vi "Remove Sequence Element.vi"(8 "error in (no error)":errorcluster, 10 "Name":string, 11 "Sequence Controller in":refnum<class "Sequence Controller.lvclass">) -> (0 "error out":errorcluster, 3 "Sequence Controller out":refnum<class "Sequence Controller.lvclass">)   [LabVIEW 2016, in "Sequence Controller.lvclass"]
uses:
  Sequence Controller.lvclass
  C:/Program Files/National Instruments/LabVIEW 2016/vi.lib/ActorFramework/Actor/Actor.lvclass
  <vilib>/ActorFramework/Actor/Actor.lvclass/Actor.ctl
  Sequence Controller.lvclass/Sequence Controller.ctl
  Template Module Messages/Stop Object Msg/Stop Object Msg.lvclass/Stop Object Msg.ctl
  <vilib>/ActorFramework/Message Enqueuer/Message Enqueuer.lvclass/Message Enqueuer.ctl
  <vilib>/ActorFramework/Message Enqueuer/Enqueue.vi
  Template Module Messages/Stop Object Msg/Stop Object Msg.lvclass
  C:/Program Files/National Instruments/LabVIEW 2016/vi.lib/ActorFramework/Message/Message.lvclass
  <vilib>/ActorFramework/Message Priority Queue/Priority Enqueue.vi
  <vilib>/ActorFramework/Actor/Actor.lvclass
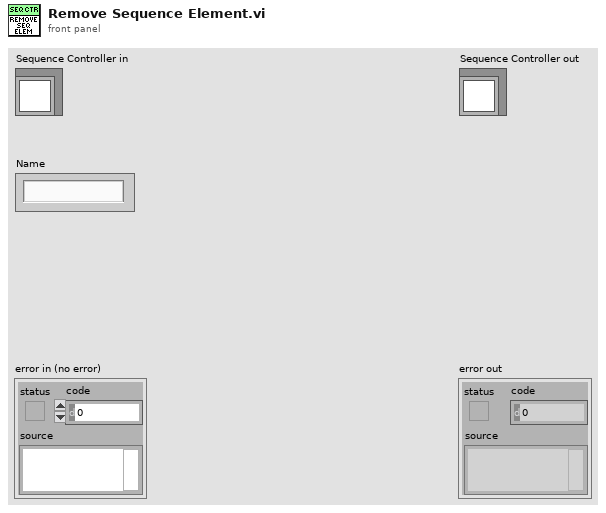
[diagram p1: front panel]
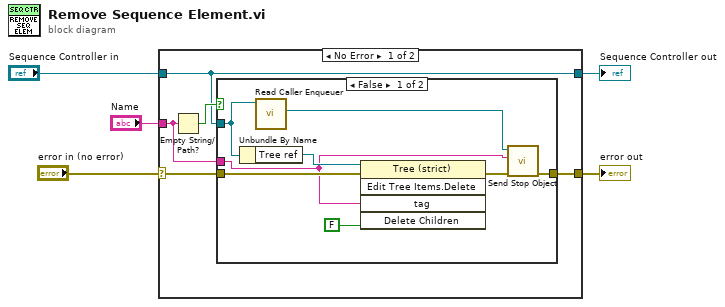
[diagram p0: block diagram]
diagram:
  n1 = case shown="No Error" "error in (no error)" {
    selector: "error in (no error)" -> [w7 w21]
    tunnel: [w6 w21] -> w4
    tunnel: [w9 w20] -> w2
    tunnel: "Sequence Controller in" -> [w9 w20]
    tunnel: "Name" -> [w8 _]
    frame No Error {
      n2 = Empty String/Path?(string/path=w8) -> (empty?=w10:bool)
      n3 = case shown="False" w10 {
        tunnel: w9 -> [w18 _]
        tunnel: w8 -> [w11 _]
        tunnel: w7 -> [w15 w19]
        tunnel: [w12 w19] -> w6
        frame False {
          n4 = Unbundle By Name(w18) -> ("Tree ref"=w17:refnum<vi>)
          n5 = call <vilib>:"Read Caller Enqueuer.vi"("Actor"=w18) -> ("Caller Enqueuer"=w14:refnum<class "Message Enqueuer.lvclass">)  [unwired: 10 in]
          n6 = invoke class="Tree (strict)" method="Edit Tree Items.Delete"(reference=w17, error in=w15, "tag"=w11, "Delete Children"=FALSE ("Delete Children?")) -> (error out=w13:errorcluster)  [unwired: 1 in, 4 out]
          n7 = call "Send Stop Object.vi"("error in (no error)"=w13, "Name"=w11, "Message Enqueuer"=w14) -> ("error out"=w12:errorcluster)  [unwired: 7 in, 1 out]
        }
        frame True {
        }
      }
    }
    frame Error {
    }
  }
  "error out" <- w4
  "Sequence Controller out" <- w2
